vi "Waveform to Display Array.vi"(8 "error in (no error)":errorcluster, 11 "Waveform Chart":dynamicdata(waveform)) -> (0 "error out":errorcluster, 3 "Array":T1[](array[typedef]))   [LabVIEW 2014, in "Display Panel.lvlib" / "Display Panel V3.lvclass"]
uses:
  Display Panel V3.lvclass
  Controls/Numeric Indicator.ctl
  <vilib>/express/express shared/transition.llb/Dynamic To Waveform Array.vi
  <vilib>/express/express signal manip/GetorSetDDTAttributes/Get DDT Attributes/Get DDT Properties.xnode
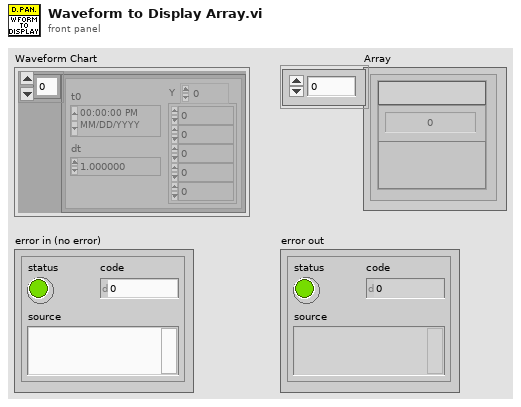
[diagram p1: front panel]
types:
  T1 = typedef "Numeric Indicator.ctl" = cluster{"Value":dbl, "Name":string, "Graph Button":bool}
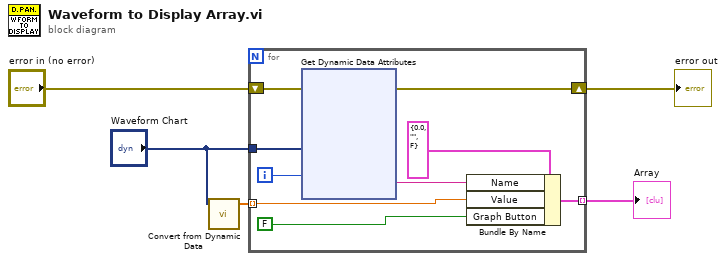
[diagram p0: block diagram]
diagram:
  n1 = call "Convert from Dynamic Data"("Dynamic Data Type"="Waveform Chart") -> ("Array"=w1:dbl[])  [unwired: 3 in]
  n2 = for {
    tunnel: w1 -> [w13] mode=indexing
    tunnel: "Waveform Chart" -> [w12]
    tunnel: [w10] -> w3 mode=indexing
    shift-right: [w6] -> w5
    shift-left: "error in (no error)" -> [w7]
    i -> [w9]
    n3 = xnode "Get Dynamic Data Attributes"("Signals In"=w12, "Signal Index"=w9, "error in"=w7) -> ("Signal Name"=w11:string, "error out"=w6:errorcluster)  [unwired: 1 out]
    n4 = Bundle By Name(cluster=T1 {"Value"=0.0, "Name"="", "Graph Button"=FALSE} ("Cluster 2"), "Name"=w11, "Value"=w13, "Graph Button"=FALSE) -> (w10:T1)
  }
  "error out" <- w5
  "Array" <- w3
